vi "send_internal_trigger.vi"(7 "ensure unique insertion?":bool, 8 "error in (no error)":errorcluster, 10 "trigger":T1, 11 "DL090202ScanHead in":refnum<class "ScanHeadDL090202.lvclass">) -> (0 "error out":errorcluster, 3 "DL090202ScanHead out":refnum<class "ScanHeadDL090202.lvclass">, 4 "# elements in queue":i32, 6 "freshly inserted?":bool)   [LabVIEW 2010, in "ScanHeadDL090202.lvclass"]
uses:
  ScanHeadDL090202.lvclass
  internal_trigger_enum.ctl
  common/classes/GenericToplevelComponent/GenericToplevelComponent/trigger_type_enum.ctl
  common/classes/ErrorController/ErrorController/class_data.vi
  common/classes/ErrorController/ErrorController/ErrorController.lvclass
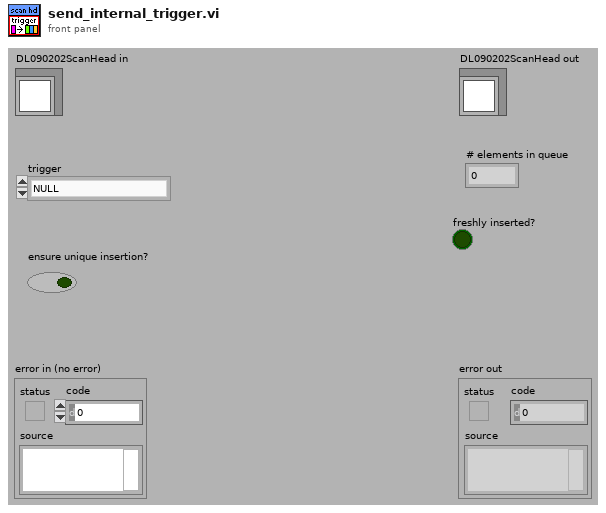
[diagram p1: front panel]
types:
  T1 = typedef "ScanHeadDL090202.lvclass/internal_trigger_enum.ctl" = enum16{"NULL", "initialise", "terminate", "start scanning", "stop scanning", "scale", "rotate", "tilt", "translate", "update modifiers", "fetch trajectory", "set run mode", "initialise scanners", "terminate scanners", "generate trajectory", "prepare writing", "write"}
  T2 = typedef "trigger_type_enum.ctl" = enum8{"external", "internal", "common"}
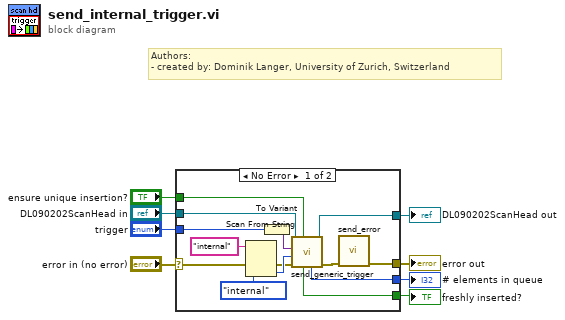
[diagram p0: block diagram]
diagram:
  # "Authors: \n- created by: Dominik Langer, University of Zurich, Switzerland"
  n1 = case shown="No Error" "error in (no error)" {
    selector: "error in (no error)" -> [w10 w24]
    tunnel: [w22 w24] -> w7
    tunnel: [w19 w23] -> w3
    tunnel: "DL090202ScanHead in" -> [w17 w23]
    tunnel: "ensure unique insertion?" -> [w18 _]
    tunnel: "trigger" -> [w14 _]
    tunnel: [w16 _] -> w2
    tunnel: [w15 _] -> w1
    frame No Error {
      n2 = Scan From String(input string="internal", error in=w10, default 1=trigger_type_enum."internal" ("trigger type")) -> (error out=w9:errorcluster, output 1=w13:T2)  [unwired: 2 in, 2 out]
      n3 = To Variant(anything=w14) -> (Variant=w21:variant)
      n4 = call-dynamic "send_generic_trigger.vi"("ensure unique insertion?"=w18, "error in (no error)"=w9, "trigger type"=w13, "trigger variant"=w21, "GenericToplevelComponent in"=w17) -> ("error out"=w20:errorcluster, "GenericToplevelComponent out"=w19:refnum<class "ScanHeadDL090202.lvclass">, "# elements in queue"=w16:i32, "freshly inserted?"=w15:bool)  [unwired: 3 in]
      n5 = call "send_error.vi"("error in (no error)"=w20) -> ("error out"=w22:errorcluster)  [unwired: 10 in]
    }
    frame Error {
    }
  }
  "error out" <- w7
  "DL090202ScanHead out" <- w3
  "# elements in queue" <- w2
  "freshly inserted?" <- w1
